vi "Updated Motion Metric.vi"() -> ()   [LabVIEW 2014]
uses:
  <vilib>/vision/NI_Vision_Development_Module.lvlib
panel:
  out "x displacement":sgl[](array[numeric])
  out "All":cluster{"x":sgl, "y":sgl, sgl}[](graph)
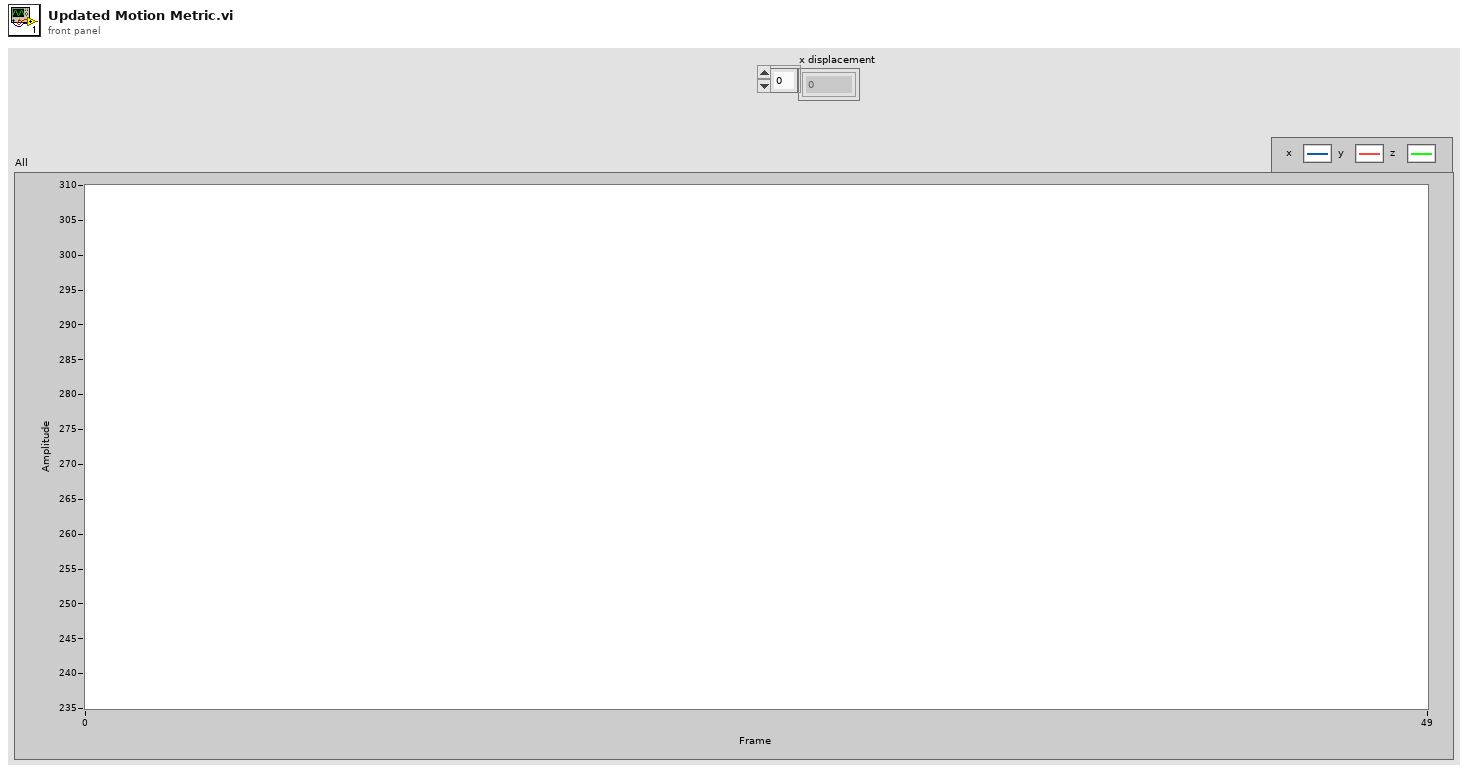
[diagram p1: front panel]
types:
  T1 = typedef "IMAQ Rectangle" = cluster{"Left":i32, "Top":i32, "Right":i32, "Bottom":i32, "Rotation":dbl}
  T2 = typedef "AviRefnum.ctl" = refnum<k1>
  T3 = typedef "IMAQ Image.ctl" = refnum<image>
  T4 = typedef "ROI Descriptor" = cluster{"Global Rectangle":i32[], "Contours":cluster{"ID":enum32{"External", "Internal"}, "Type":u32, "Coordinates":i32[]}[]}
  T5 = cluster{"Position":cluster{"x":sgl, "y":sgl}, "Angle":sgl, "Scale":sgl, "Score":sgl, "Bounding Box":cluster{"x":sgl, "y":sgl}[]}[]
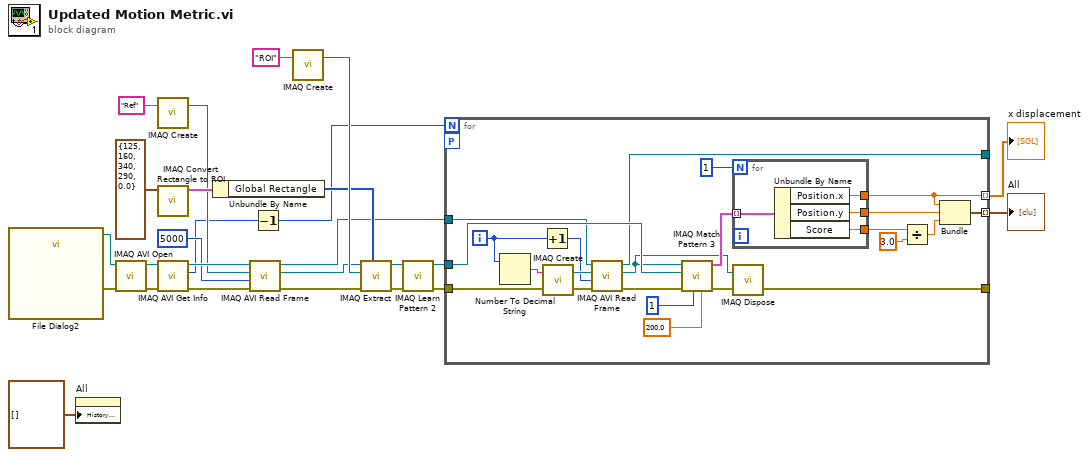
[diagram p0: block diagram]
diagram:
  n1 = call "File Dialog2"() -> ("selected path"=w7:path, "error out"=w8:errorcluster)  [unwired: 12 in, 2 out]
  n2 = property on="All" class="WFChart (strict)"("History Data"=cluster{"x":sgl, "y":sgl, "Score":sgl}[] []) -> ()  [unwired: 2 in, 2 out]
  n3 = call "IMAQ AVI Open"("error in (no error)"=w8, "AVI Path"=w7) -> ("error out"=w14:errorcluster, "Avi Refnum"=w12:T2)  [unwired: 8 in]
  n4 = call "IMAQ Create"("Image Name"="Ref") -> ("New Image"=w10:T3)  [unwired: 4 in, 1 out]
  n5 = call "IMAQ Convert Rectangle to ROI"("Rectangle"=T1 {"Left"=125, "Top"=160, "Right"=340, "Bottom"=290, "Rotation"=0.0}) -> ("ROI Descriptor"=w18:T4)  [unwired: 8 in, 1 out]
  n6 = call "IMAQ AVI Get Info"("error in (no error)"=w14, "Avi Refnum"=w12) -> ("error out"=w13:errorcluster, "Number of Frames"=w3:u32, "Avi Refnum (duplicate)"=w11:T2)  [unwired: 5 in, 2 out]
  n7 = Unbundle By Name(w18) -> ("Global Rectangle"=w17:i32[])
  n8 = call "IMAQ AVI Read Frame"("error in (no error)"=w13, "Frame Number"=u32 5000, "Image"=w10, "Avi Refnum"=w11) -> ("error out"=w6:errorcluster, "Image Out"=w5:T3, "Avi Refnum (duplicate)"=w4:T2)  [unwired: 4 in, 1 out]
  n9 = Decrement(x=w3) -> (x-1=w2:u32)
  n10 = call "IMAQ Create"("Image Name"="ROI") -> ("New Image"=w25:T3)  [unwired: 4 in, 1 out]
  n11 = call "IMAQ Extract"("Optional Rectangle"=w17, "error in (no error)"=w6, "Image Dst"=w25, "Image Src"=w5) -> ("error out"=w23:errorcluster, "Image Dst Out"=w21:T3)  [unwired: 6 in]
  n12 = call "IMAQ Learn Pattern 2"("error in (no error)"=w23, "Image"=w21) -> ("error out"=w22:errorcluster, "Template Image Out"=w20:T3)  [unwired: 8 in]
  n13 = for {
    N: w2 -> [_]
    tunnel: w4 -> [w29]
    tunnel: w22 -> [w44]
    tunnel: w20 -> [w45]
    tunnel: [w39] -> w15 mode=indexing
    workers-P: _ -> [_]
    tunnel: [w35] -> _
    tunnel: [w28] -> _
    tunnel: [w27] -> w1 mode=indexing
    i -> [w37]
    n14 = Number To Decimal String(number=w37) -> (decimal integer string=w36:string)  [unwired: 1 in]
    n15 = Increment(x=w37) -> (x+1=w30:i32)
    n16 = call "IMAQ Create"("Image Name"=w36, "error in (no error)"=w44) -> ("New Image"=w31:T3, "error out"=w34:errorcluster)  [unwired: 3 in]
    n17 = call "IMAQ AVI Read Frame"("error in (no error)"=w34, "Frame Number"=w30, "Image"=w31, "Avi Refnum"=w29) -> ("error out"=w33:errorcluster, "Image Out"=w32:T3, "Avi Refnum (duplicate)"=w28:T2)  [unwired: 4 in, 1 out]
    n18 = call "IMAQ Match Pattern 3"("Minimum Match Score"=sgl 200.0, "Number of Matches Requested"=1, "error in (no error)"=w33, "Template Image"=w45, "Image"=w32) -> ("error out"=w38:errorcluster, "Matches"=w47:T5)  [unwired: 4 in, 1 out]
    n19 = for {
      N: 1 -> [_]
      tunnel: w47 -> [w53] mode=indexing
      tunnel: [w52] -> w27
      tunnel: [w51] -> w43
      tunnel: [w50] -> w40
      n20 = Unbundle By Name(w53) -> ("Position.x"=w52:sgl, "Position.y"=w51:sgl, "Score"=w50:sgl)
    }
    n21 = call "IMAQ Dispose"("Image"=w32, "error in (no error)"=w38) -> ("error out"=w35:errorcluster)  [unwired: 4 in]
    n22 = Divide(x=w40, y=sgl 3.0) -> (x/y=w41:sgl)
    n23 = Bundle("x"=w27, "y"=w43, w41) -> (w39:cluster{"x":sgl, "y":sgl, sgl})  [unwired: 1 in]
  }
  "All" <- w15
  "x displacement" <- w1
